vi "PIO.Read Byte Array.vi"(8 "error in (no error)":errorcluster, 9 "count":u32, 10 "offset":u32 format="%.0x", 11 "GE 5565PIORC in":refnum<class "GE 5565PIORC.lvclass">) -> (0 "error out":errorcluster, 2 "bytes read":u8[](array[numeric]), 3 "GE 5565PIORC out":refnum<class "GE 5565PIORC.lvclass">)   [LabVIEW 2016, in "GE 5565PIORC.lvclass"]
uses:
  GE 5565PIORC.lvclass
  GE 5565PIORC.lvclass/GE 5565PIORC.ctl
  Change Endianness (1D U32).vi
  Change Endianness (U32).vi
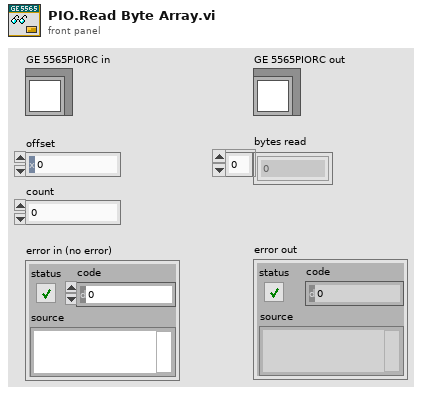
[diagram p1: front panel]
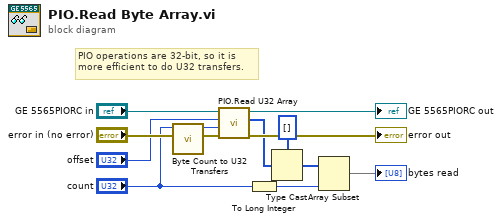
[diagram p0: block diagram]
diagram:
  # "PIO operations are 32-bit, so it is more efficient to do U32 transfers."
  n1 = call "Byte Count to U32 Transfers.vi"("bytes to transfer"="count") -> ("U32 transfers"=w7:u32)  [unwired: 9 in, 1 out]
  n2 = call "PIO.Read U32 Array.vi"("error in (no error)"="error in (no error)", "count"=w7, "offset"="offset", "GE 5565PIORC in"="GE 5565PIORC in") -> ("error out"=→"error out":errorcluster, "values"=w1:u32[], "GE 5565PIORC out"=→"GE 5565PIORC out":refnum<class "GE 5565PIORC.lvclass">)  [unwired: 5 in]
  n3 = To Long Integer(number="count") -> (32bit integer=w2:i32)
  n4 = Type Cast(type=u8[] [], x=w1) -> (*(type *) &x=w5:u8[])
  n5 = Array Subset(array=w5, length=w2) -> (→"bytes read":u8[])  [unwired: 1 in]
